vi "SetExposure.vi"(8 "error in (no error)":errorcluster, 10 "Exposure(ms)":dbl, 11 "Inovance_Camera in":refnum<class "Inovance_Camera.lvclass">) -> (0 "error out":errorcluster, 3 "Inovance_Camera out":refnum<class "Inovance_Camera.lvclass">)   [LabVIEW 2023, in "Inovance_Camera.lvlib" / "Inovance_Camera.lvclass"]
uses:
  Inovance_Camera.lvclass
  <vilib>/userDefined/High Color/IMAQdx.ctl
  Inovance_Camera.lvclass/Inovance_Camera.ctl
  Inovance_Camera.lvlib
  Interfaces/AbstractInstrumentClasses/Cameras_LV/CameraComm Messages/Exposure Set Msg/Exposure Set Msg.lvclass
  <vilib>/ActorFramework/Actor/Actor.lvclass
  C:/Program Files/National Instruments/LabVIEW 2023/vi.lib/ActorFramework/Actor/Actor.lvclass
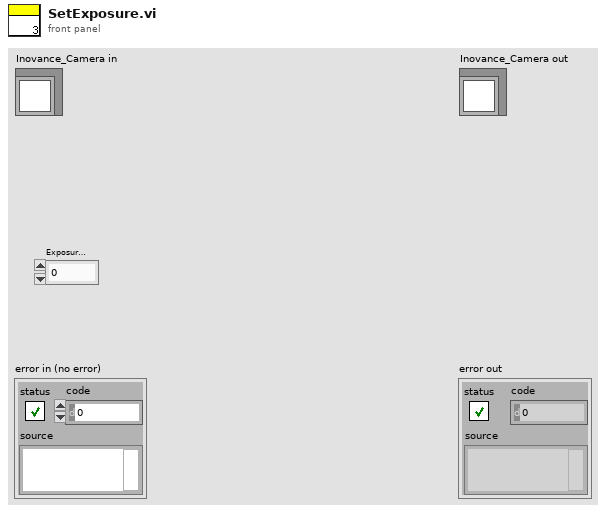
[diagram p1: front panel]
types:
  T1 = typedef "IMAQdx.ctl" = refnum<k21>
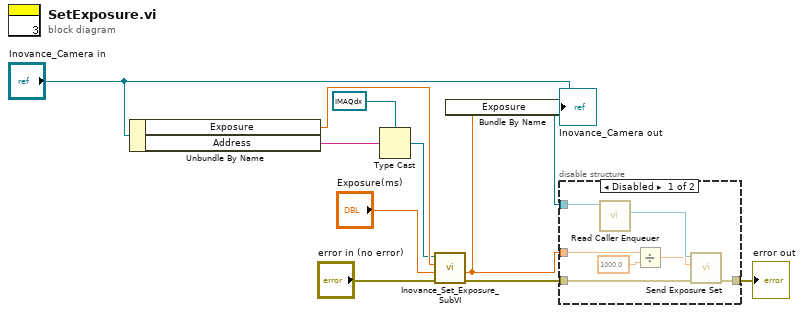
[diagram p0: block diagram]
diagram:
  n1 = Unbundle By Name("Inovance_Camera in") -> ("Exposure"=w10:dbl, "Address"=w2:string)
  n2 = Type Cast(type=T1 refnum ("Inovance Address"), x=w2) -> (*(type *) &x=w3:T1)
  n3 = call "Inovance_Set_Exposure_SubVI.vi"("error in (no error)"="error in (no error)", "Exposure"="Exposure(ms)", "OldVal"=w10, "Refnum in"=w3) -> ("error out"=w7:errorcluster, "Exposure Out"=w1:dbl)  [unwired: 5 in, 1 out]
  n4 = Bundle By Name(cluster="Inovance_Camera in", "Exposure"=w1) -> (w4:refnum<class "Inovance_Camera.lvclass">)
  "Inovance_Camera out" <- w4
  n5 = disable-structure shown="Disabled" {
    disable-tunnel: w7 -> [w17 w19]
    disable-tunnel: [w16 w19] -> w6
    disable-tunnel: w4 -> [w15 _]
    disable-tunnel: w1 -> [w14 _]
    frame Disabled {
      n6 = call <vilib>:"Read Caller Enqueuer.vi"("Actor"=w15) -> ("Caller Enqueuer"=w18:refnum<class "Message Enqueuer.lvclass">)  [unwired: 10 in]
      n7 = Divide(x=w14, y=1000.0) -> (x/y=w12:dbl)
      n8 = call "Send Exposure Set.vi"("error in (no error)"=w17, "Exposure(ms)"=w12, "Message Enqueuer"=w18) -> ("error out"=w16:errorcluster)  [unwired: 7 in, 1 out]
    }
    frame Enabled {
    }
  }
  "error out" <- w6
